vi "test json to variant array.vi"(8 "error in (no error)":errorcluster) -> (0 "error out":errorcluster)   [LabVIEW 2019, in "labview_json_tests.lvlib"]
uses:
  labview_json_tests.lvlib
  lib/labview_json.lvlib
panel:
  out "Variant out":variant
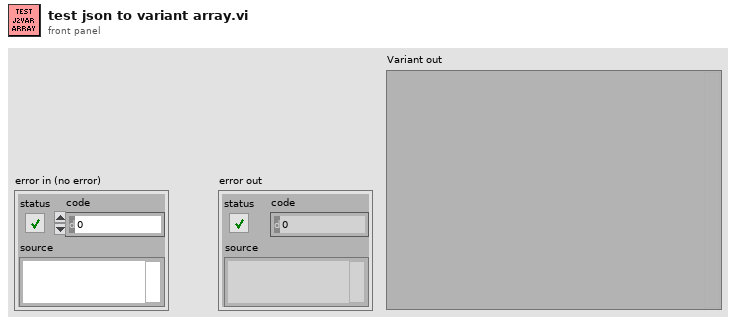
[diagram p1: front panel]
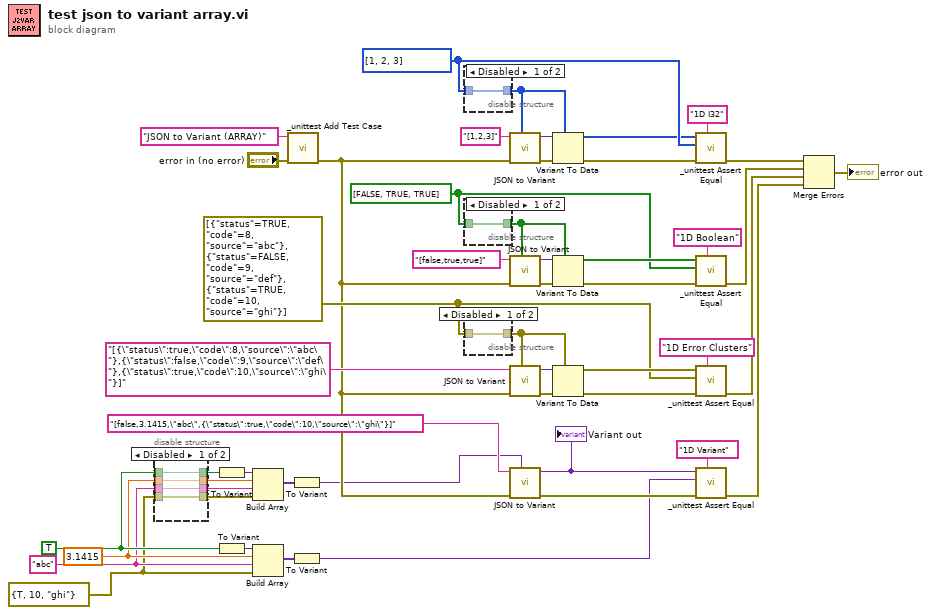
[diagram p0: block diagram]
diagram:
  w4 = errorcluster {"status"=TRUE, "code"=10, "source"="ghi"} ("error out")
  w6 = "abc"
  w8 = 3.1415
  w10 = TRUE
  w21 = errorcluster[] [{"status"=TRUE, "code"=8, "source"="abc"}, {"status"=FALSE, "code"=9, "source"="def"}, {"status"=TRUE, "code"=10, "source"="ghi"}]
  w31 = bool[] [FALSE, TRUE, TRUE] ("Array")
  w41 = i32[] [1, 2, 3] ("Array")
  n1 = disable-structure shown="Disabled" {
    disable-tunnel: w10 -> [w54 _]
    disable-tunnel: [w54 _] -> w9
    disable-tunnel: w8 -> [w53 _]
    disable-tunnel: [w53 _] -> w7
    disable-tunnel: w6 -> [w52 _]
    disable-tunnel: [w52 _] -> w5
    disable-tunnel: w4 -> [w51 _]
    disable-tunnel: [w51 _] -> w3
    frame Disabled {
    }
    frame Enabled {
    }
  }
  n2 = To Variant(anything=w9) -> (Variant=w11:variant)
  n3 = To Variant(anything=w10) -> (Variant=w16:variant)
  n4 = Build Array(w11, w7, w5, w3) -> (w12:variant[])
  n5 = Build Array(w16, w8, w6, w4) -> (w15:variant[])
  n6 = call "_unittest Add Test Case.vi"("error in (no error)"="error in (no error)", "Test Case"="JSON to Variant (ARRAY)") -> ("error out"=w19:errorcluster)  [unwired: 9 in]
  n7 = To Variant(anything=w12) -> (Variant=w2:variant)
  n8 = To Variant(anything=w15) -> (Variant=w1:variant)
  n9 = disable-structure shown="Disabled" {
    disable-tunnel: [w55 _] -> w40
    disable-tunnel: w41 -> [w55 _]
    frame Disabled {
    }
    frame Enabled {
    }
  }
  n10 = disable-structure shown="Disabled" {
    disable-tunnel: [w56 _] -> w37
    disable-tunnel: w31 -> [w56 _]
    frame Disabled {
    }
    frame Enabled {
    }
  }
  n11 = disable-structure shown="Disabled" {
    disable-tunnel: [w57 _] -> w24
    disable-tunnel: w21 -> [w57 _]
    frame Disabled {
    }
    frame Enabled {
    }
  }
  n12 = call "JSON to Variant.vi"("Variant Type"=w40, "error in (no error)"=w19, "JSON"="[1,2,3]") -> ("error out"=w46:errorcluster, "Variant out"=w42:variant)  [unwired: 7 in]
  n13 = call "JSON to Variant.vi"("Variant Type"=w37, "error in (no error)"=w19, "JSON"="[false,true,true]") -> ("error out"=w33:errorcluster, "Variant out"=w36:variant)  [unwired: 7 in]
  n14 = call "JSON to Variant.vi"("Variant Type"=w24, "error in (no error)"=w19, "JSON"="[{\"status\":true,\"code\":8,\"source\":\"abc\"},{\"status\":false,\"code\":9,\"source\":\"def\"},{\"status\":true,\"code\":10,\"source\":\"ghi\"}]") -> ("error out"=w28:errorcluster, "Variant out"=w25:variant)  [unwired: 7 in]
  n15 = call "JSON to Variant.vi"("Variant Type"=w2, "error in (no error)"=w19, "JSON"="[false,3.1415,\"abc\",{\"status\":true,\"code\":10,\"source\":\"ghi\"}]") -> ("error out"=w13:errorcluster, "Variant out"=w14:variant)  [unwired: 7 in]
  "Variant out" <- w14
  n16 = Variant To Data(error in=w46, type=w40, Variant=w42) -> (data=w39:i32[], error out=w43:errorcluster)
  n17 = Variant To Data(error in=w33, type=w37, Variant=w36) -> (data=w38:bool[], error out=w35:errorcluster)
  n18 = Variant To Data(error in=w28, type=w24, Variant=w25) -> (data=w23:errorcluster[], error out=w26:errorcluster)
  n19 = call "_unittest Assert Equal.vi"("Message"="1D I32", "error in (no error)"=w43, "Expected Value"=w41, "Actual Value"=w39) -> ("error out"=w48:errorcluster)  [unwired: 7 in]
  n20 = call "_unittest Assert Equal.vi"("Message"="1D Boolean", "error in (no error)"=w35, "Expected Value"=w31, "Actual Value"=w38) -> ("error out"=w30:errorcluster)  [unwired: 7 in]
  n21 = call "_unittest Assert Equal.vi"("Message"="1D Error Clusters", "error in (no error)"=w26, "Expected Value"=w21, "Actual Value"=w23) -> ("error out"=w22:errorcluster)  [unwired: 7 in]
  n22 = call "_unittest Assert Equal.vi"("Message"="1D Variant", "error in (no error)"=w13, "Expected Value"=w1, "Actual Value"=w14) -> ("error out"=w18:errorcluster)  [unwired: 7 in]
  n23 = Merge Errors(w48, w30, w22, w18) -> (→"error out":errorcluster)
